vi "MOKE_Teperature and FIeld Sweep_1022D.vi"() -> ()   [LabVIEW 2022 SP3]
uses:
  <vilib>/Analysis/baseanly.llb/Mean (DBL).vi
  <vilib>/Utility/file.llb/Write Delimited Spreadsheet (DBL).vi
  <vilib>/Analysis/NI_AALBase.lvlib
panel:
  out "Rh1 B/A v F":cluster{dbl[], dbl[]}(graph)
  in  "?":bool
  out "Temperature Status":i32(ring) items=["TemperatureUnknown"=0, "Stable"=1, "Tracking"=2, "Near"=5, "Chasing"=6, "Filling"=7, "Standby"=10, "Disabled"=13, "ImpedanceNotFunction"=14, "TempFailure"=15]
  out "Field Status":i32(ring) items=["MagnetUnknown"=0, "StablePersistent"=1, "WarmingSwitch"=2, "CoolingSwitch"=3, "StableDriven"=4, "Iterating"=5, "Charging"=6, "Discharging"=7, "CurrentError"=8, "MagnetFailure"=15]
  out "Field":dbl
  out "Temperature":dbl
  in  "Initialize":bool
  in  "System Stablization (s)":dbl=0.1 format="%#_13g"
  in  "Low Value (Oe)":dbl=-30000.0
  in  "High Value (Oe)":dbl=30000.0
  in  "Sweep Field Approach":i32(ring) items=["Linear", "NoOvershoot", "Oscillate"]
  in  "Sweep F Rate (Oe/s)":dbl=200.0 format="%#_13g"
  in  "Sweep F mode":i32(ring) items=["Persistent", "Driven"]
  in  "Set Fixed T":dbl=2.0
  in  "Fixed Temperature Approach":i32(ring)=1 items=["FastSettle", "NoOvershoot"]
  in  "FIxed T  Rate (K/min)":dbl=20.0
  out "PhaseA-F":cluster{dbl[], dbl[]}(graph)
  out "RA-F":cluster{dbl[], dbl[]}(graph)
  out "Phaseh1B-F":cluster{dbl[], dbl[]}(graph)
  out "Rh1B-F":cluster{dbl[], dbl[]}(graph)
  out "phase B 2":dbl
  in  "Phase B 2":u16(ring)=3 items=["X", "Y", "R", "Theta", "Frequency", "Noise", "Xh1", "Yh1", "Rh1", "Theta h1", "Xh2", "Yh2", "Rh2", "Theta h2"]
  out "phase A 2":dbl
  in  "Phase A 2":u16(ring)=3 items=["X", "Y", "R", "Theta", "Frequency", "Noise", "Xh1", "Yh1", "Rh1", "Theta h1", "Xh2", "Yh2", "Rh2", "Theta h2"]
  out "para1 Measurement (mV) 2":dbl=1.49013e-07
  in  "F Clear Plot A":bool
  in  "Parameter A 2":u16(ring)=2 items=["X", "Y", "R", "Theta", "Frequency", "Noise", "Xh1", "Yh1", "Rh1", "Theta h1", "Xh2", "Yh2", "Rh2", "Theta h2"]
  out "para2 Measurement (uV) 2":dbl=1.49013e-07
  in  "F Clear Plot B":bool
  in  "Parameter B 2":u16(ring)=2 items=["X", "Y", "R", "Theta", "Frequency", "Noise", "Xh1", "Yh1", "Rh1", "Theta h1", "Xh2", "Yh2", "Rh2", "Theta h2"]
  out "Field Setting":dbl format="%#_13g"
  out "Fixed Temperature":dbl
  out "Measured Field":dbl
  out "Field Status":i32(ring) items=["MagnetUnknown"=0, "StablePersistent"=1, "WarmingSwitch"=2, "CoolingSwitch"=3, "StableDriven"=4, "Iterating"=5, "Charging"=6, "Discharging"=7, "CurrentError"=8, "MagnetFailure"=15]
  out "Temperature Status":i32(ring) items=["TemperatureUnknown"=0, "Stable"=1, "Tracking"=2, "Near"=5, "Chasing"=6, "Filling"=7, "Standby"=10, "Disabled"=13, "ImpedanceNotFunction"=14, "TempFailure"=15]
  out "Measuring F":bool
  in  "Step(Oe)":i32=2000
  out "F loop run":i32
  out "Temperature Status":i32(ring) items=["TemperatureUnknown"=0, "Stable"=1, "Tracking"=2, "Near"=5, "Chasing"=6, "Filling"=7, "Standby"=10, "Disabled"=13, "ImpedanceNotFunction"=14, "TempFailure"=15]
  out "Field Status":i32(ring) items=["MagnetUnknown"=0, "StablePersistent"=1, "WarmingSwitch"=2, "CoolingSwitch"=3, "StableDriven"=4, "Iterating"=5, "Charging"=6, "Discharging"=7, "CurrentError"=8, "MagnetFailure"=15]
  out "Fixed Field":dbl
  out "Measured Temperature":dbl
  in  "Delay(T/F)":dbl=3000.0
  in  "Set FIxed F (Oe)":dbl format="%#_13g"
  in  "Fixed Field Approach":i32(ring) items=["Linear", "NoOvershoot", "Oscillate"]
  in  "FIxed F Rate (Oe/s)":dbl=100.0 format="%#_13g"
  in  "Fixed F mode":i32(ring) items=["Persistent", "Driven"]
  in  "Sweep Temperature Approach":i32(ring)=1 items=["FastSettle", "NoOvershoot"]
  in  "Sweep T  Rate (K/min)":dbl=10.0
  in  "Sweep T/F":bool
  in  "Remote":bool=TRUE
  in  "IP Address":string="169.254.170.239"
  out "Measuring T":bool
  in  "A Sine Output Amplitude (V)":sgl=0.1
  in  "path (folder + filename)":string="C:\\Users\\Public\\OneDrive\\Desktop\\MOKE program\\sweep files"
  in  "LOCKIN address":refnum<visa-resource-name>="COM3"
  out "PhaseA-T":cluster{dbl[], dbl[]}(graph)
  out "RA-T":cluster{dbl[], dbl[]}(graph)
  out "Phaseh1-T":cluster{dbl[], dbl[]}(graph)
  out "Rh1B-T":cluster{dbl[], dbl[]}(graph)
  out "phase B":dbl
  in  "Phase B":u16(ring)=9 items=["X", "Y", "R", "Theta", "Frequency", "Noise", "Xh1", "Yh1", "Rh1", "Theta h1", "Xh2", "Yh2", "Rh2", "Theta h2"]
  out "phase A":dbl
  in  "Phase A":u16(ring)=3 items=["X", "Y", "R", "Theta", "Frequency", "Noise", "Xh1", "Yh1", "Rh1", "Theta h1", "Xh2", "Yh2", "Rh2", "Theta h2"]
  out "para1 Measurement (mV)":dbl=1.49013e-07
  in  "T Clear Plot A":bool
  in  "Parameter A":u16(ring)=2 items=["X", "Y", "R", "Theta", "Frequency", "Noise", "Xh1", "Yh1", "Rh1", "Theta h1", "Xh2", "Yh2", "Rh2", "Theta h2"]
  out "para2 Measurement (uV)":dbl=1.49013e-07
  in  "T Clear Plot B":bool
  in  "Parameter B":u16(ring)=8 items=["X", "Y", "R", "Theta", "Frequency", "Noise", "Xh1", "Yh1", "Rh1", "Theta h1", "Xh2", "Yh2", "Rh2", "Theta h2"]
  out "Temperature Setting":dbl format="%#_13g"
  in  "Save data or not":bool=TRUE
  in  "Step(K)":i32=10
  out "T loop run":i32
  in  "B frequency":dbl=267.7 format="%#_13g"
  in  "B Input Connection (0: Single-Ended)":u16(ring)=1 items=["Single-Ended Voltage", "Differential Voltage", "1 MOhm Current Gain", "100 MOhm Current Gain"]
  in  "B harmonic 1":u8=2
  in  "B harmonic 2":u8=3
  in  "B reference Manual Phase":dbl=-59.75
  in  "auto phase B":bool=TRUE
  in  "B Sample time (s)":dbl=0.001 min=0.001 max=100.0 step=0.001
  in  "B Sensitivity":u16(ring)=20 items=["1 nV/fA", "2 nV/fA", "5 nV/fA", "10 nV/fA", "20 nV/fA", "50 nV/fA", "100 nV/fA", "200 nV/fA", "500 nV/fA", "1 uV/pA", "2 uV/pA", "5 uV/pA", "10 uV/pA", "20 uV/pA", "50 uV/pA", "100 uV/pA", "200 uV/pA", "500 uV/pA", "1 mV/nA", "2 mV/nA", "5 mV/nA", "10 mV/nA", "20 mV/nA", "50 mV/nA", "100 mV/nA", "200 mV/nA", "500 mV/nA", "1 V/uA"]
  in  "Enable Sync Filter B (open when f<200Hz)":bool
  in  "B Time Constant":u8(ring)=9 items=["10 us", "30 us", "100 us", "300 us", "1 ms", "3 ms", "10 ms", "30 ms", "100 ms", "300 ms", "1 s", "3 s", "10 s", "30 s", "100 s", "300 s", "1 ks", "3 ks"]
  in  "B Reference Source":u8(ring) items=["External", "Internal", "Internal Sweep", "Channel-A"]
  in  "B Low Pass Filter Slope":u8(ring)=2 items=["6 dB/oct", "12 dB/oct", "18 db/oct", "24 dB/oct"]
  in  "A frequency":dbl=267.7 format="%#_13g"
  in  "A Input Connection (0: Single-Ended)":u16(ring)=1 items=["Single-Ended Voltage", "Differential Voltage", "1 MOhm Current Gain", "100 MOhm Current Gain"]
  in  "A harmonic 1":u8=2
  in  "A harmonic 2":u8=3
  in  "A reference Manual Phase":dbl=-59.75
  in  "auto phase A":bool=TRUE
  in  "A Reference Source":u8(ring)=1 items=["External", "Internal", "Internal Sweep"]
  in  "A Sample time (s)":dbl=0.001 min=0.001 max=100.0 step=0.001
  in  "A Time Constant":u8(ring)=9 items=["10 us", "30 us", "100 us", "300 us", "1 ms", "3 ms", "10 ms", "30 ms", "100 ms", "300 ms", "1 s", "3 s", "10 s", "30 s", "100 s", "300 s", "1 ks", "3 ks"]
  in  "Enable Sync Filter A (open when f<200Hz)":bool
  in  "A Sensitivity":u16(ring)=20 items=["1 nV/fA", "2 nV/fA", "5 nV/fA", "10 nV/fA", "20 nV/fA", "50 nV/fA", "100 nV/fA", "200 nV/fA", "500 nV/fA", "1 uV/pA", "2 uV/pA", "5 uV/pA", "10 uV/pA", "20 uV/pA", "50 uV/pA", "100 uV/pA", "200 uV/pA", "500 uV/pA", "1 mV/nA", "2 mV/nA", "5 mV/nA", "10 mV/nA", "20 mV/nA", "50 mV/nA", "100 mV/nA", "200 mV/nA", "500 mV/nA", "1 V/uA"]
  in  "A Low Pass Filter Slope":u8(ring)=2 items=["6 dB/oct", "12 dB/oct", "18 db/oct", "24 dB/oct"]
  in  "stabilization(S)":dbl=0.1 format="%#_13g"
  in  "High Value (K)":dbl=300.0
  in  "Low Value (K)":dbl=2.0
  in  "loop #":i32=1
  # "Status"
  # "Lock-in Setting"
  # "Channel A"
  # "Channel B"
  # "Sweep F Mesurement"
  # "Temprature and Field Setting"
  # "Sweep T Mesurement"
  # "Sweep F"
  # "Sweep T"
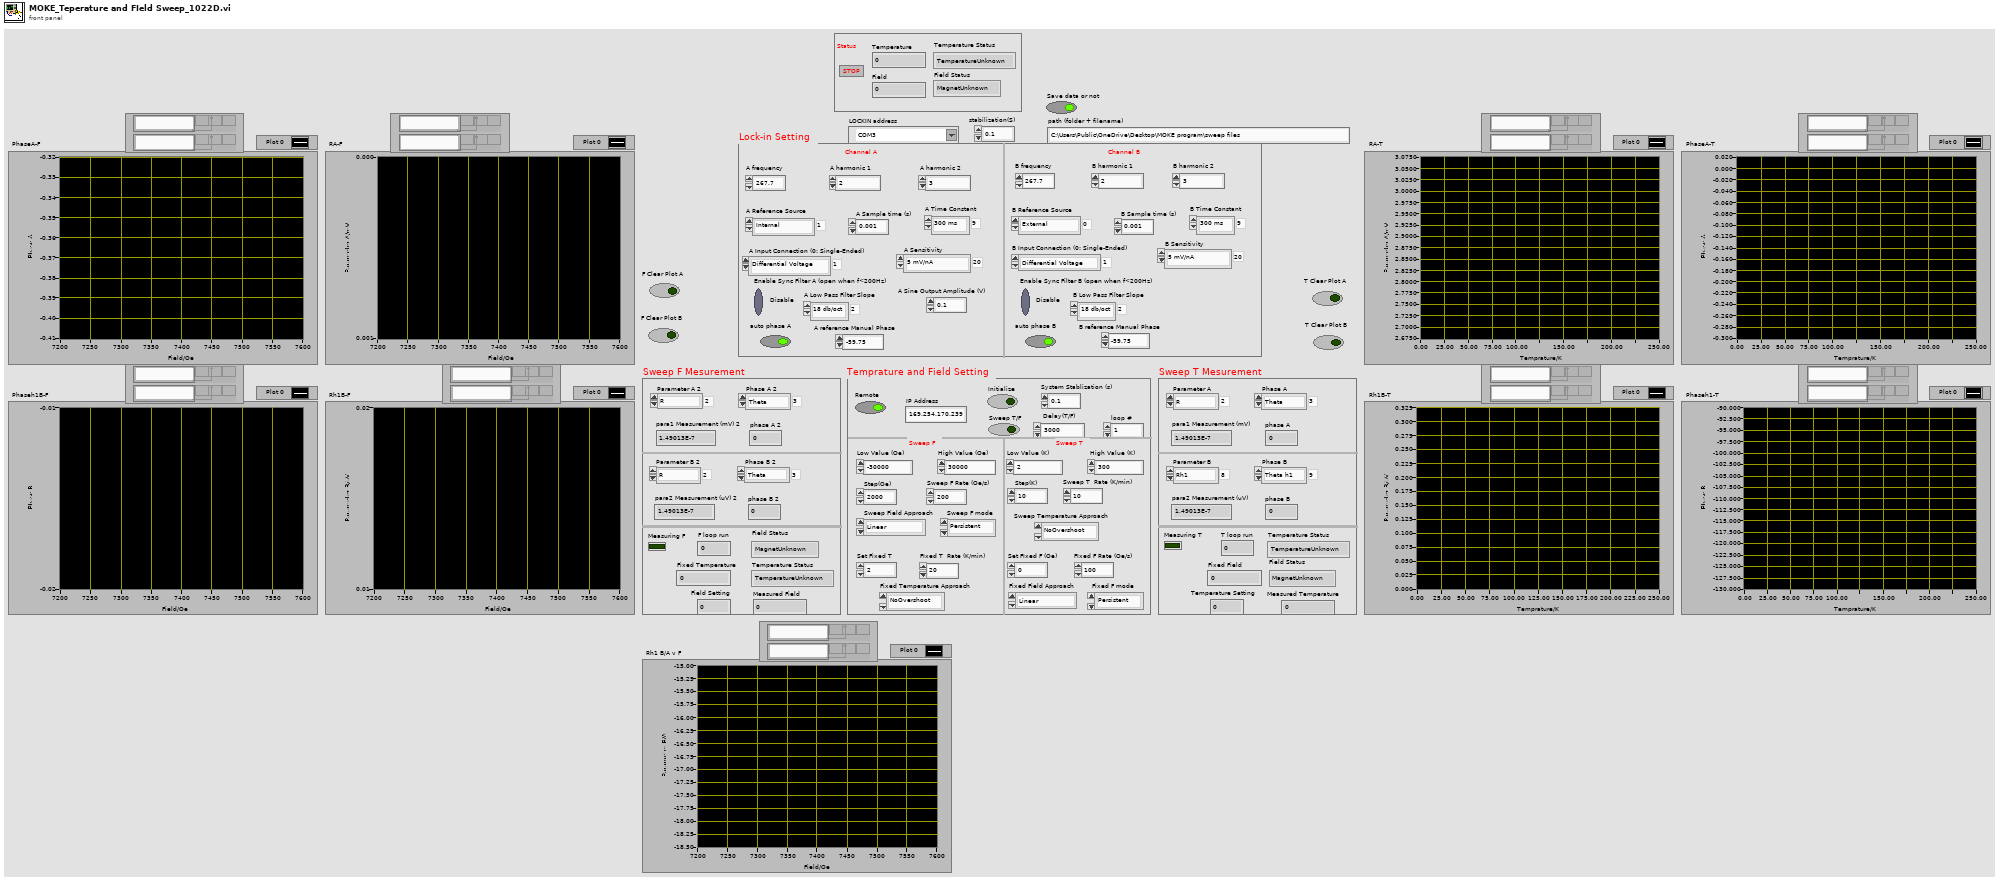
[diagram p1: front panel]
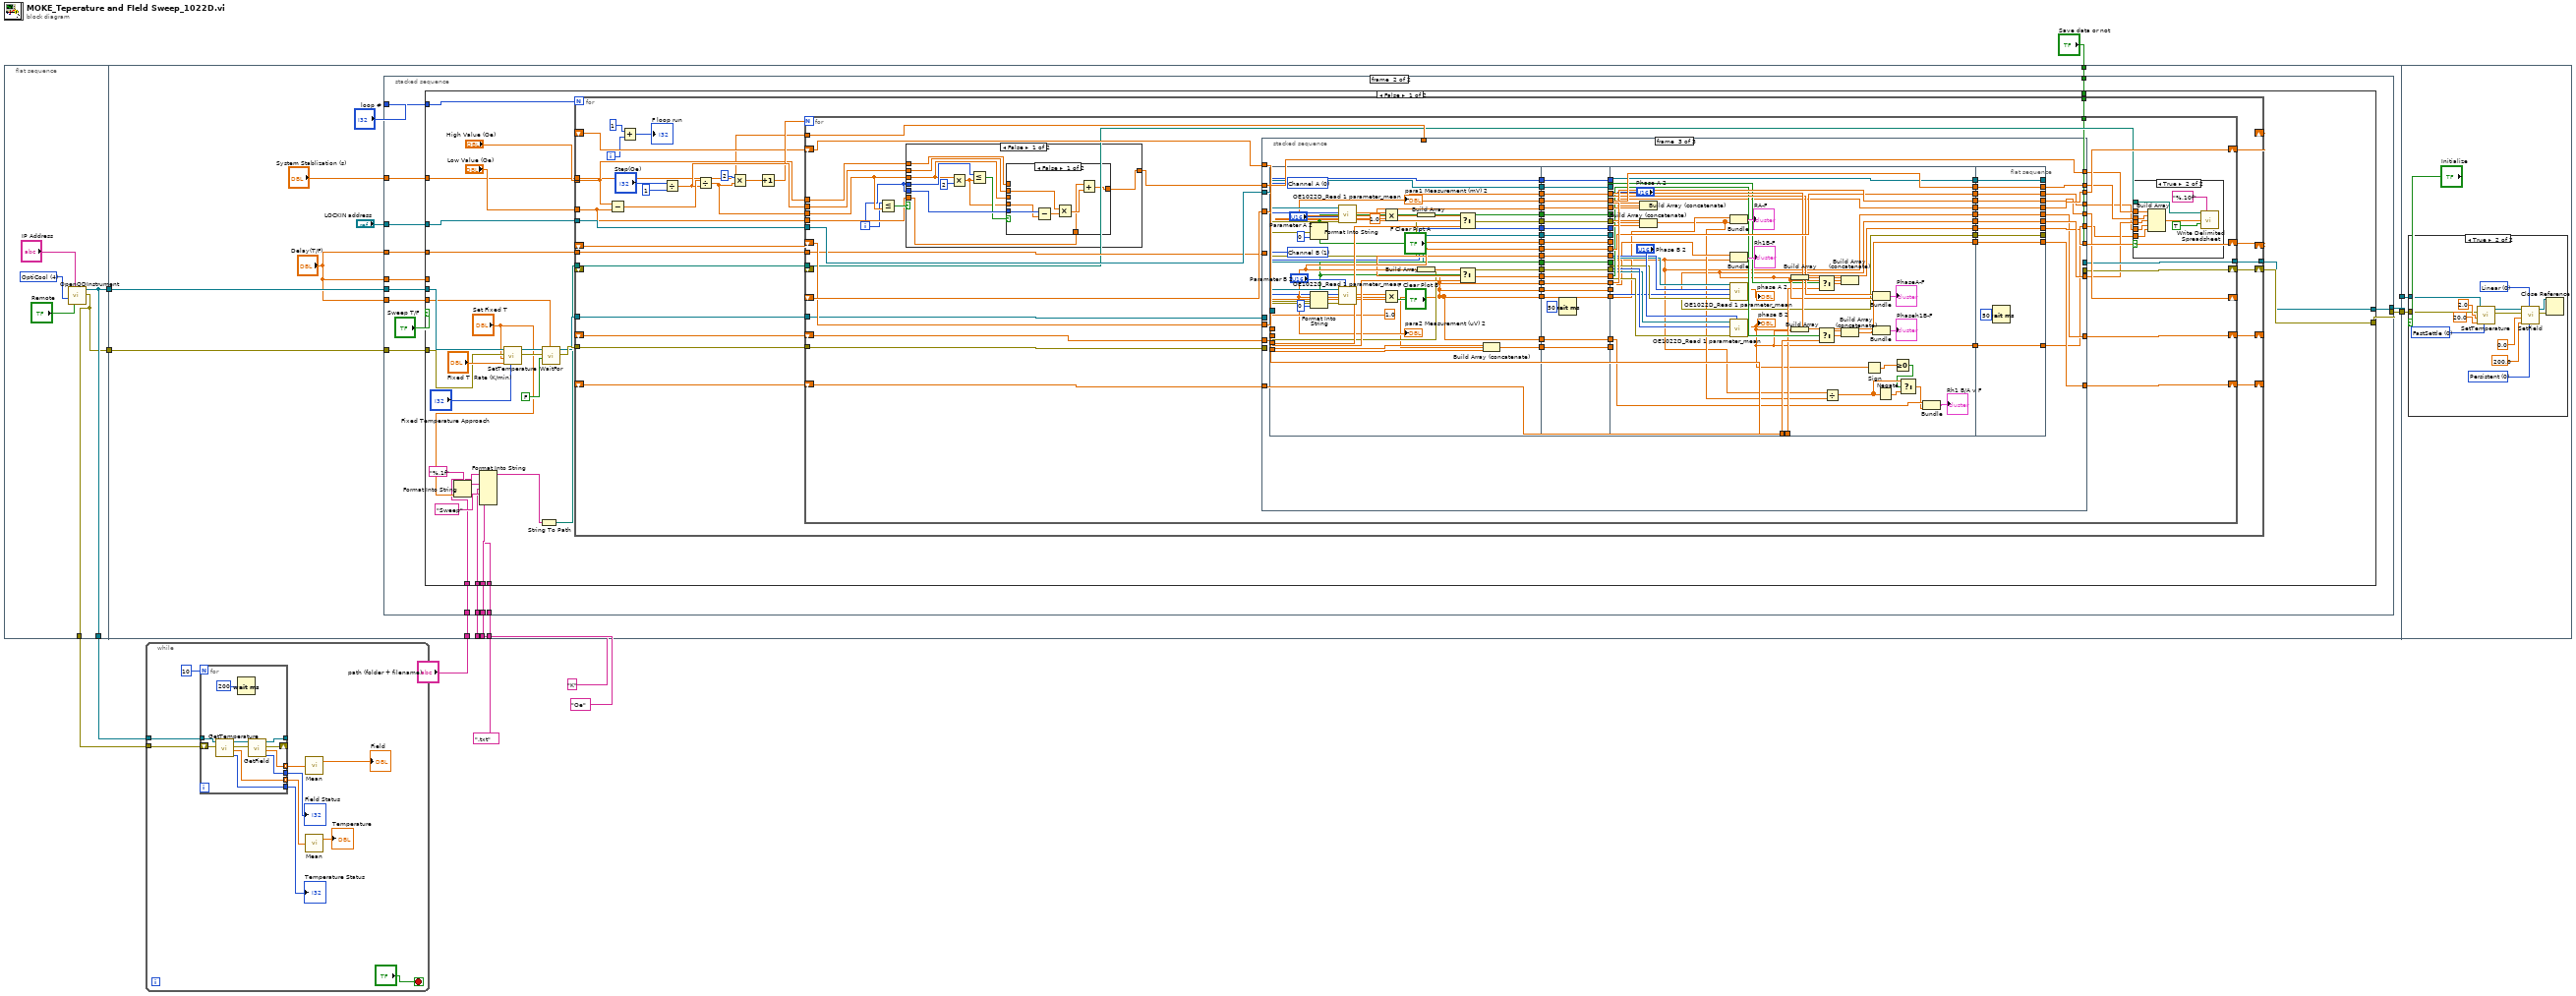
[diagram p0: block diagram]
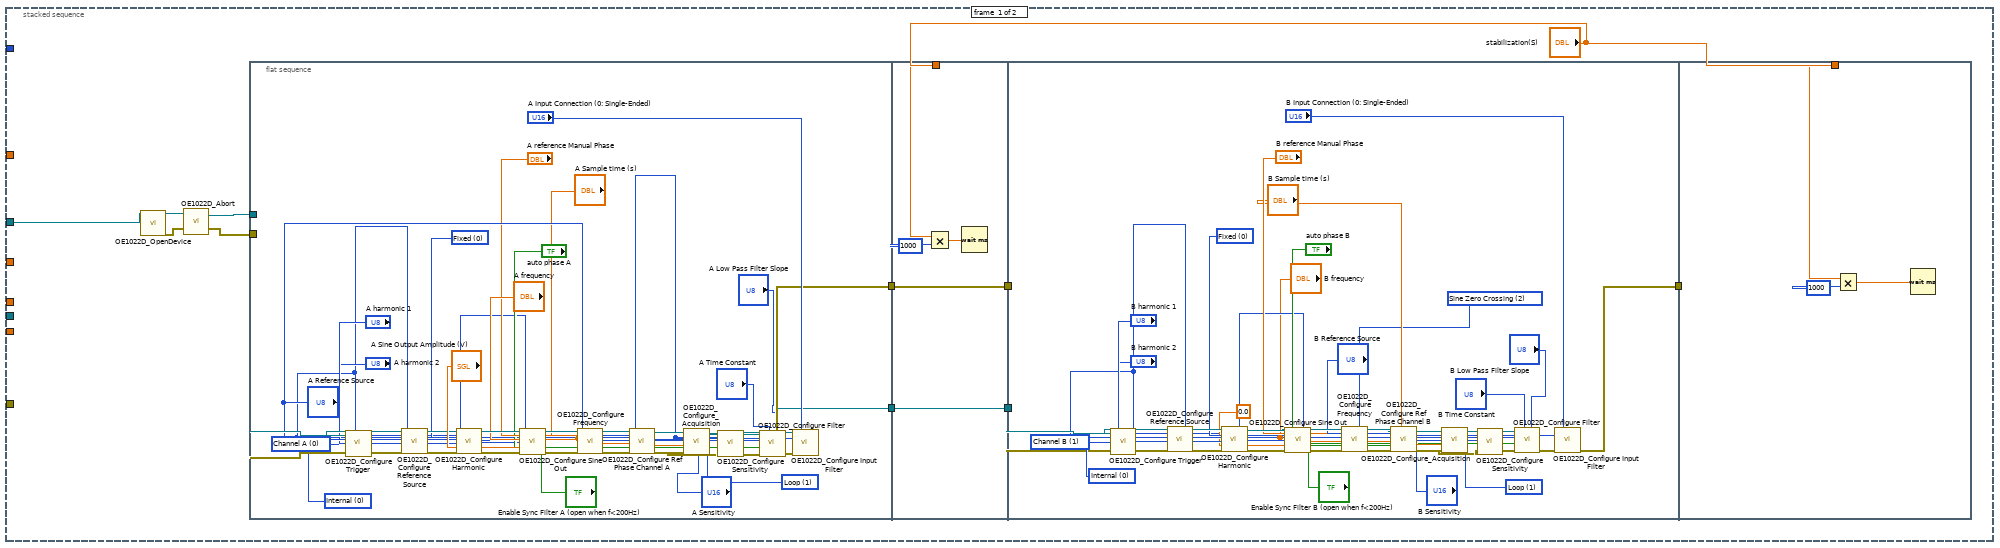
[diagram p2: hidden frame]
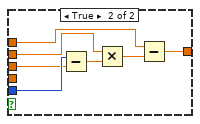
[diagram p4: hidden frame]
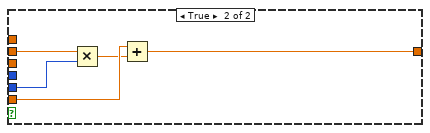
[diagram p5: hidden frame]
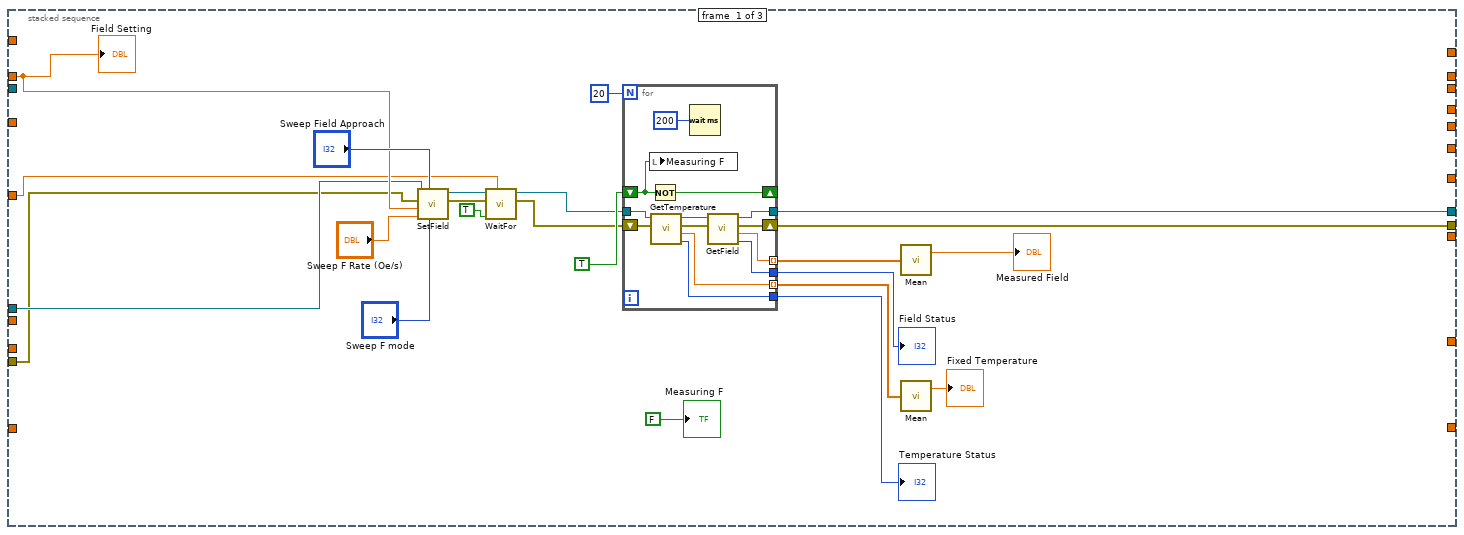
[diagram p6: hidden frame]
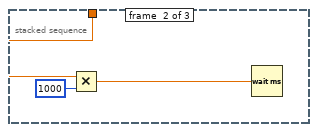
[diagram p7: hidden frame]
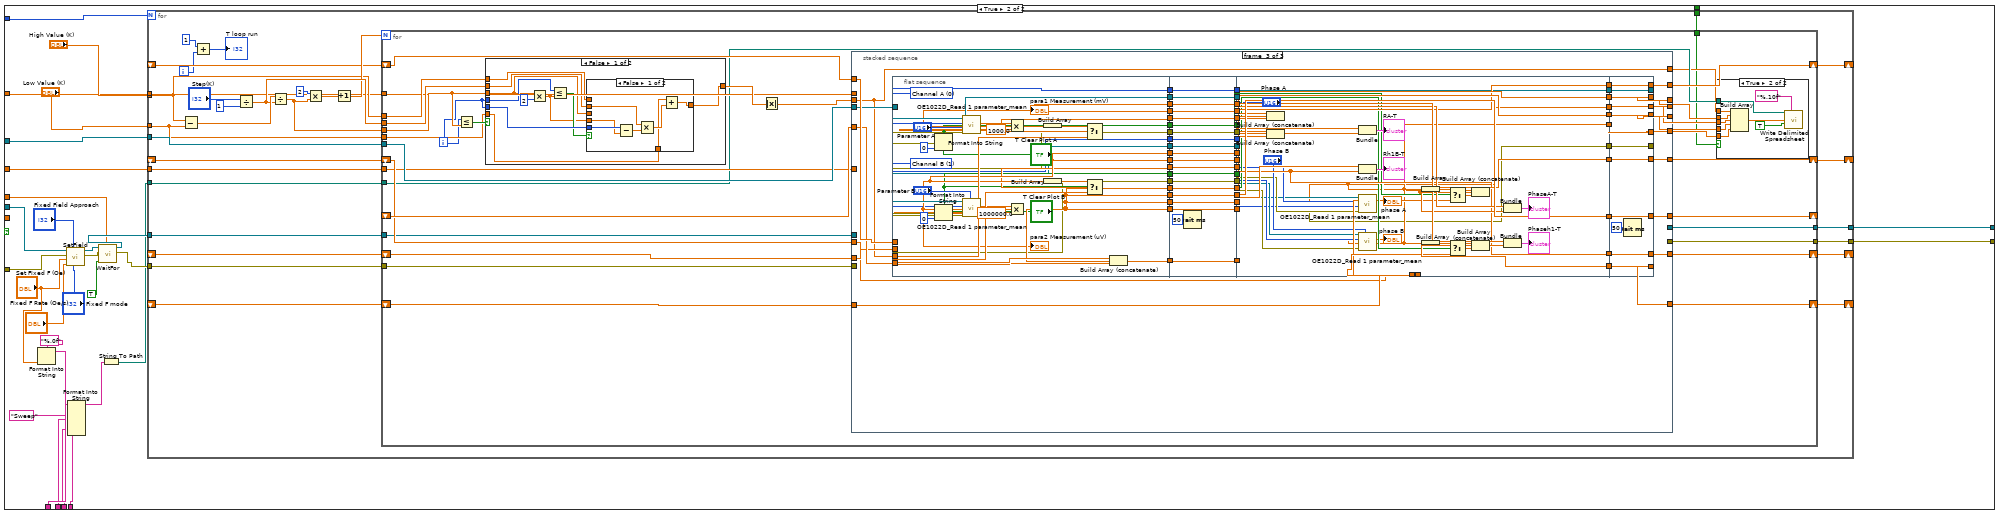
[diagram p8: hidden frame]
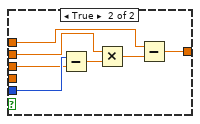
[diagram p10: hidden frame]
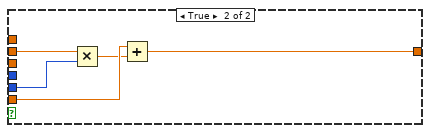
[diagram p11: hidden frame]
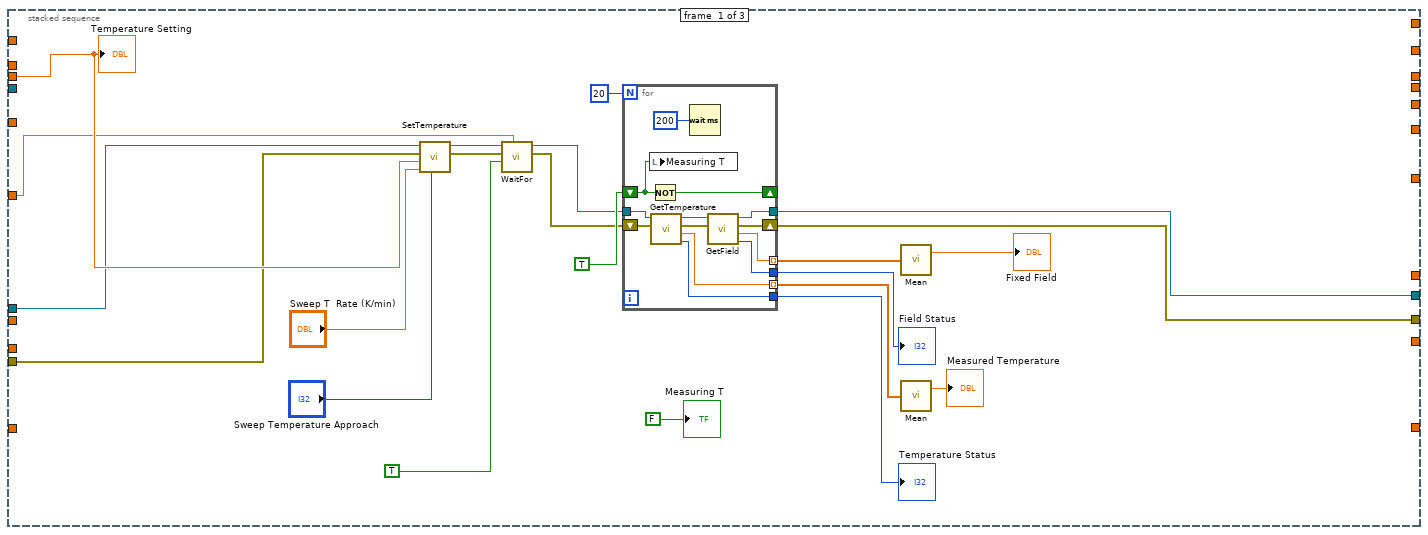
[diagram p12: hidden frame]
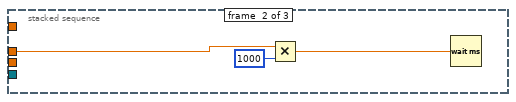
[diagram p13: hidden frame]
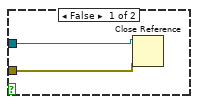
[diagram p14: hidden frame]
diagram:
  n1 = flat-sequence {
    tunnel: [w13] -> w11
    tunnel: [w12] -> w10
    tunnel: [w13] -> w3
    tunnel: [w12] -> w2
    tunnel: w11 -> [w27]
    tunnel: w10 -> [w26]
    tunnel: "path (folder + filename)" -> [w24]
    tunnel: "Oe" -> [w23]
    tunnel: "K" -> [w22]
    tunnel: ".txt" -> [w21]
    tunnel: [w19] -> w5
    tunnel: [w18] -> w4
    tunnel: "Save data or not" -> [w17]
    tunnel: w5 -> [w819]
    tunnel: w4 -> [w818]
    frame #0 {
      w14 = 4 items=["PPMS", "VersaLab", "DynaCool", "SVSM", "OptiCool"] ("InstrumentType")
      n2 = call "OpenQDInstrument.vi"("Remote"="Remote", "IP Address"="IP Address", "InstrumentType"=w14) -> ("error out"=w12:errorcluster, "Instrument Ref"=w13:refnum<k24>)  [unwired: 5 in]
    }
    frame #1 {
      n3 = stacked-sequence {
        tunnel: "LOCKIN address" -> [w32 w141]
        tunnel: "loop #" -> [_ w140]
        tunnel: w27 -> [_ w138]
        tunnel: w26 -> [_ w137]
        tunnel: "Delay(T/F)" -> [_ w136]
        tunnel: "Delay(T/F)" -> [_ w135]
        tunnel: "Delay(T/F)" -> [_ w134]
        tunnel: w24 -> [_ w133]
        tunnel: w23 -> [_ w132]
        tunnel: w22 -> [_ w131]
        tunnel: w21 -> [_ w130]
        tunnel: "System Stablization (s)" -> [_ w129]
        tunnel: [_ w128] -> w19
        tunnel: [_ w127] -> w18
        tunnel: w17 -> [_ w126]
        frame #0 {
          n4 = call "OE1022D_OpenDevice.vi"("VISA resource name"=w32) -> ("VISA资源名称输出"=w31:refnum<visa-resource-name>, "错误输出"=w33:errorcluster)  [unwired: 17 in]
          n5 = call "OE1022D_Abort.vi"("error in (no error)"=w33, "VISA resource name"=w31) -> ("error out"=w38:errorcluster, "VISA resource name out"=w39:refnum<visa-resource-name>)
          n6 = flat-sequence {
            tunnel: w39 -> [w79]
            tunnel: [w67] -> w37
            tunnel: w38 -> [w78]
            tunnel: [w55] -> w35
            tunnel: w37 -> [w84]
            tunnel: [w84] -> w36
            tunnel: w35 -> [w83]
            tunnel: [w83] -> w34
            tunnel: "stabilization(S)" -> [w80]
            tunnel: w36 -> [w105]
            tunnel: [w104] -> w40
            tunnel: w34 -> [w103]
            tunnel: w40 -> [_]
            tunnel: "stabilization(S)" -> [w123]
            frame #0 {
              w41 = u8 1 items=["Single", "Loop"] ("Sample Mode (Single/Loop)")
              w54 = u8 0 items=["Fixed", "Linear", "Log"] ("SineOut Mode")
              w56 = u16 0 items=["Internal", "External"] ("Trigger Source (0: Internal)")
              w45 = u8 0 items=["Channel A", "Channel B"] ("OE1022D A/B")
              n7 = call "OE1022D_Configure Trigger.vi"("Trigger Source (0: Internal)"=w56, "error in (no error)   2"=w78, "OE1022D A/B"=w45, "VISA resource name   2"=w79) -> ("error out   2"=w72:errorcluster, "VISA resource name out   2"=w73:refnum<visa-resource-name>)
              n8 = call "OE1022D_Configure Reference Source.vi"("VISA resource name"=w73, "OE1022D A/B"=w45, "Reference Source"="A Reference Source", "error in (no error)"=w72) -> ("VISA resource name out"=w71:refnum<visa-resource-name>, "error out"=w69:errorcluster)  [unwired: 14 in]
              n9 = call "OE1022D_Configure Harmonic.vi"("VISA resource name"=w71, "OE1022D A/B"=w45, "Harmonic 1"="A harmonic 1", "Harmonic 2"="A harmonic 2", "error in (no error)"=w69) -> ("VISA resource name out"=w70:refnum<visa-resource-name>, "error out"=w68:errorcluster)  [unwired: 13 in]
              n10 = call "OE1022D_Configure Sine Out.vi"("VISA resource name"=w70, "SineOut Mode"=w54, "OE1022D A/B"=w45, "Sine Output Amplitude (V)"="A Sine Output Amplitude (V)", "error in (no error)"=w68) -> ("VISA resource name out"=w76:refnum<visa-resource-name>, "error out"=w75:errorcluster)  [unwired: 9 in]
              n11 = call "OE1022D_Configure Frequency.vi"("VISA resource name"=w76, "OE1022D A/B"=w45, "Internal Frequency(Hz)"="A frequency", "error in (no error)"=w75) -> ("VISA resource name out"=w66:refnum<visa-resource-name>, "error out"=w63:errorcluster)  [unwired: 14 in]
              n12 = call "OE1022D_Configure Ref Phase Channel A.vi"("VISA resource name"=w66, "Reference Source"="A Reference Source", "Internal Frequency(Hz)"="A frequency", "Auto Phase (T: Enabled)"="auto phase A", "error in (no error)"=w63, "Manual Phase  (degree)"="A reference Manual Phase") -> ("VISA resource name out"=w65:refnum<visa-resource-name>, "error out"=w64:errorcluster)  [unwired: 12 in]
              n13 = call "OE1022D_Configure_Acquisition.vi"("VISA resource name"=w65, "OE1022D A/B"=w45, "Sample time (s)"="A Sample time (s)", "error in (no error)"=w64, "Sample Mode (Single/Loop)"=w41) -> ("VISA resource name out"=w48:refnum<visa-resource-name>, "error out"=w47:errorcluster)  [unwired: 3 in]
              n14 = call "OE1022D_Configure Sensitivity.vi"("VISA resource name"=w48, "OE1022D A/B"=w45, "Sensitivity"="A Sensitivity", "error in (no error)"=w47) -> ("VISA resource name out"=w52:refnum<visa-resource-name>, "error out"=w51:errorcluster)  [unwired: 14 in]
              n15 = call "OE1022D_Configure Filter.vi"("Low Pass Filter Slope (1: 12dB/oct)"="A Low Pass Filter Slope", "Time Constant (8: 100ms)"="A Time Constant", "error in (no error)"=w51, "Enable Sync Filter (F: Disable)"="Enable Sync Filter A (open when f<200Hz)", "OE1022D A/B"=w45, "VISA resource name"=w52) -> ("error out"=w49:errorcluster, "VISA resource name out"=w50:refnum<visa-resource-name>)  [unwired: 4 in]
              n16 = call "OE1022D_Configure Input Filter.vi"("VISA resource name"=w50, "Input Source"="A Input Connection (0: Single-Ended)", "OE1022D A/B"=w45, "error in (no error)"=w49) -> ("VISA resource name out"=w55:refnum<visa-resource-name>, "error out"=w67:errorcluster)  [unwired: 10 in]
            }
            frame #1 {
              n17 = Multiply(x=w80, y=1000) -> (x*y=w82:dbl)
              n18 = Wait (ms)(milliseconds to wait=w82) -> ()  [unwired: 1 out]
            }
            frame #2 {
              w85 = u8 1 items=["Single", "Loop"] ("Sample Mode (Single/Loop)")
              w87 = u8 2 items=["TTL Pos", "TTL Neg", "Sine Zero Crossing"] ("External Ref Trigger")
              w100 = u8 0 items=["Fixed", "Linear", "Log"] ("SineOut Mode")
              w106 = u16 0 items=["Internal", "External"] ("Trigger Source (0: Internal)")
              w92 = u8 1 items=["Channel A", "Channel B"] ("OE1022D A/B")
              n19 = call "OE1022D_Configure Trigger.vi"("Trigger Source (0: Internal)"=w106, "error in (no error)   2"=w105, "OE1022D A/B"=w92, "VISA resource name   2"=w103) -> ("error out   2"=w118:errorcluster, "VISA resource name out   2"=w119:refnum<visa-resource-name>)
              n20 = call "OE1022D_Configure Reference Source.vi"("VISA resource name"=w119, "OE1022D A/B"=w92, "error in (no error)"=w118) -> ("VISA resource name out"=w117:refnum<visa-resource-name>, "error out"=w115:errorcluster)  [unwired: 15 in]
              n21 = call "OE1022D_Configure Harmonic.vi"("VISA resource name"=w117, "OE1022D A/B"=w92, "Harmonic 1"="B harmonic 1", "Harmonic 2"="B harmonic 2", "error in (no error)"=w115) -> ("VISA resource name out"=w116:refnum<visa-resource-name>, "error out"=w114:errorcluster)  [unwired: 13 in]
              n22 = call "OE1022D_Configure Sine Out.vi"("VISA resource name"=w116, "SineOut Mode"=w100, "OE1022D A/B"=w92, "Sine Output Amplitude (V)"=sgl 0.0, "error in (no error)"=w114) -> ("VISA resource name out"=w121:refnum<visa-resource-name>, "error out"=w120:errorcluster)  [unwired: 9 in]
              n23 = call "OE1022D_Configure Frequency.vi"("VISA resource name"=w121, "OE1022D A/B"=w92, "Internal Frequency(Hz)"="B frequency", "error in (no error)"=w120) -> ("VISA resource name out"=w113:refnum<visa-resource-name>, "error out"=w110:errorcluster)  [unwired: 14 in]
              n24 = call "OE1022D_Configure Ref Phase Channel B.vi"("VISA resource name"=w113, "Reference Source"="B Reference Source", "External Ref Trigger"=w87, "Internal Frequency(Hz)"="B frequency", "Auto Phase (T: Enabled)"="auto phase B", "error in (no error)"=w110, "Manual Phase  (degree)"="B reference Manual Phase") -> ("VISA resource name out"=w112:refnum<visa-resource-name>, "error out"=w111:errorcluster)  [unwired: 11 in]
              n25 = call "OE1022D_Configure_Acquisition.vi"("VISA resource name"=w112, "OE1022D A/B"=w92, "Sample time (s)"="B Sample time (s)", "error in (no error)"=w111, "Sample Mode (Single/Loop)"=w85) -> ("VISA resource name out"=w93:refnum<visa-resource-name>, "error out"=w94:errorcluster)  [unwired: 3 in]
              n26 = call "OE1022D_Configure Sensitivity.vi"("VISA resource name"=w93, "OE1022D A/B"=w92, "Sensitivity"="B Sensitivity", "error in (no error)"=w94) -> ("VISA resource name out"=w97:refnum<visa-resource-name>, "error out"=w96:errorcluster)  [unwired: 14 in]
              n27 = call "OE1022D_Configure Filter.vi"("Low Pass Filter Slope (1: 12dB/oct)"="B Low Pass Filter Slope", "Time Constant (8: 100ms)"="B Time Constant", "error in (no error)"=w96, "Enable Sync Filter (F: Disable)"="Enable Sync Filter B (open when f<200Hz)", "OE1022D A/B"=w92, "VISA resource name"=w97) -> ("error out"=w95:errorcluster)  [unwired: 4 in, 1 out]
              n28 = call "OE1022D_Configure Input Filter.vi"("Input Source"="B Input Connection (0: Single-Ended)", "OE1022D A/B"=w92, "error in (no error)"=w95) -> ("error out"=w104:errorcluster)  [unwired: 11 in, 1 out]
            }
            frame #3 {
              n29 = Multiply(x=w123, y=1000) -> (x*y=w125:dbl)
              n30 = Wait (ms)(milliseconds to wait=w125) -> ()  [unwired: 1 out]
            }
          }
        }
        frame #1 {
          n31 = case shown="False" "Sweep T/F" {
            tunnel: w141 -> [w169 w513]
            tunnel: w140 -> [w170 w512]
            tunnel: w138 -> [w161 w508]
            tunnel: w137 -> [w162 w507]
            tunnel: w136 -> [_ w501]
            tunnel: w135 -> [w168 w500]
            tunnel: w134 -> [w160 _]
            tunnel: w133 -> [w151 w495]
            tunnel: w132 -> [w150 w491]
            tunnel: w131 -> [w149 w492]
            tunnel: w130 -> [w148 w490]
            tunnel: w129 -> [w145 w487]
            tunnel: [w144 w486] -> w128
            tunnel: [w143 w485] -> w127
            tunnel: w126 -> [w142 w484]
            frame False {
              n32 = Format Into String(format string="%.1f", "Set Fixed T") -> (resulting string=w154:string)  [unwired: 2 in, 1 out]
              n33 = Format Into String(initial string=w151, w154, w149, "Sweep", w150, w148) -> (resulting string=w155:string)  [unwired: 2 in, 1 out]
              n34 = call "SetTemperature.vi"("Approach"="Fixed Temperature Approach", "Rate"="FIxed T  Rate (K/min)", "Temperature"="Set Fixed T", "error in (no error)"=w162, "Instrument Ref In"=w161) -> ("error out"=w163:errorcluster, "Instrument Ref Out"=w164:refnum<k24>)  [unwired: 2 in, 1 out]
              n35 = String To Path(string=w155) -> (path=w152:path)
              n36 = call "WaitFor.vi"("Delay"=w160, "Wait For Temperature"=FALSE ("WaitForTemperature"), "error in (no error)"=w163, "Instrument Ref In"=w164) -> ("error out"=w159:errorcluster, "Instrument Ref Out"=w158:refnum<k24>)  [unwired: 6 in]
              n37 = for {
                N: w170 -> [_]
                tunnel: w169 -> [w200]
                tunnel: "Low Value (Oe)" -> [w194]
                tunnel: "High Value (Oe)" -> [w184]
                tunnel: w152 -> [w193]
                shift-right: [w189] -> _
                shift-left: _ -> [w188]
                shift-right: [w183] -> _
                shift-left: _ -> [w182]
                shift-right: [w181] -> _
                shift-left: _ -> [w180]
                shift-right: [w179] -> _
                shift-left: _ -> [w178]
                tunnel: w158 -> [w177]
                tunnel: w159 -> [w176]
                tunnel: w168 -> [w175]
                tunnel: w145 -> [w174]
                shift-right: [w173] -> w144
                shift-left: _ -> [_]
                tunnel: [w172] -> w143
                tunnel: w142 -> [w171]
                i -> [w186]
                n38 = Subtract(x=w184, y=w194) -> (x-y=w196:dbl)
                n39 = Add(x=1, y=w186) -> (x+y=→"F loop run":i32)
                n40 = Divide(x="Step(Oe)", y=1) -> (x/y=w195:dbl)
                n41 = Divide(x=w196, y=w195) -> (x/y=w192:dbl)
                n42 = Multiply(x=2, y=w192) -> (x*y=w191:dbl)
                n43 = Increment(x=w191) -> (x+1=w190:dbl)
                n44 = for {
                  N: w190 -> [_]
                  tunnel: w200 -> [w231]
                  tunnel: w195 -> [w227]
                  shift-right: [w219] -> w189
                  shift-left: w188 -> [w230]
                  tunnel: w192 -> [w225]
                  tunnel: w194 -> [w228]
                  tunnel: w184 -> [w226]
                  tunnel: w193 -> [w207]
                  shift-right: [w218] -> _
                  shift-left: _ -> [w222]
                  shift-right: [w221] -> w183
                  shift-left: w182 -> [w220]
                  shift-right: [w217] -> w181
                  shift-left: w180 -> [w216]
                  shift-right: [w215] -> w179
                  shift-left: w178 -> [w214]
                  tunnel: w177 -> [w213]
                  tunnel: w176 -> [w212]
                  tunnel: w175 -> [w211]
                  tunnel: w174 -> [w210]
                  shift-right: [w209] -> w173
                  shift-left: _ -> [_]
                  tunnel: [w208] -> w172
                  tunnel: w171 -> [w201]
                  i -> [w224]
                  n45 = Less Or Equal?(x=w224, y=w225) -> (x <= y?=w229:bool)
                  n46 = case shown="False" w229 {
                    tunnel: w228 -> [w241 w269]
                    tunnel: w224 -> [w250 w268]
                    tunnel: w227 -> [w249 w267]
                    tunnel: [w247 w265] -> w223
                    tunnel: w226 -> [w248 _]
                    tunnel: w225 -> [w243 _]
                    tunnel: w224 -> [w246 _]
                    frame False {
                      n47 = Multiply(x=w243, y=2) -> (x*y=w242:dbl)
                      n48 = Less Or Equal?(x=w246, y=w242) -> (x <= y?=w244:bool)
                      n49 = case shown="False" w244 {
                        tunnel: w250 -> [w257 w264]
                        tunnel: w249 -> [w255 w262]
                        tunnel: w248 -> [_ w260]
                        tunnel: [w253 w259] -> w247
                        tunnel: w243 -> [_ w258]
                        tunnel: w242 -> [w252 _]
                        tunnel: w241 -> [w251 _]
                        frame False {
                          n50 = Subtract(x=w257, y=w252) -> (x-y=w256:dbl)
                          n51 = Multiply(x=w255, y=w256) -> (x*y=w254:dbl)
                          n52 = Add(x=w251, y=w254) -> (x+y=w253:dbl)
                        }
                        frame True {
                          n53 = Subtract(x=w264, y=w258) -> (x-y=w263:dbl)
                          n54 = Multiply(x=w262, y=w263) -> (x*y=w261:dbl)
                          n55 = Subtract(x=w260, y=w261) -> (x-y=w259:dbl)
                        }
                      }
                    }
                    frame True {
                      n56 = Multiply(x=w267, y=w268) -> (x*y=w266:dbl)
                      n57 = Add(x=w269, y=w266) -> (x+y=w265:dbl)
                    }
                  }
                  n58 = stacked-sequence {
                    tunnel: w231 -> [_ _ w373]
                    tunnel: w223 -> [w275 _ w372]
                    tunnel: w230 -> [_ _ w375]
                    tunnel: [_ _ w374] -> w219
                    tunnel: [_ _ w311] -> w205
                    tunnel: [_ _ w372] -> w206
                    tunnel: [_ _ w371] -> w218
                    tunnel: w222 -> [_ _ w370]
                    tunnel: [_ _ w369] -> w204
                    tunnel: [_ _ w368] -> w221
                    tunnel: w220 -> [_ _ w361]
                    tunnel: [_ _ w367] -> w217
                    tunnel: w216 -> [_ _ w362]
                    tunnel: [_ _ w366] -> w215
                    tunnel: w214 -> [_ _ w365]
                    tunnel: [_ _ w364] -> w202
                    tunnel: [_ _ w363] -> w203
                    tunnel: w213 -> [w274 _ _]
                    tunnel: w212 -> [w273 _ _]
                    tunnel: w211 -> [w272 _ _]
                    tunnel: w210 -> [_ w306 _]
                    tunnel: [w271 _ _] -> w209
                    tunnel: [w270 _ _] -> w208
                    frame #0 {
                      n59 = call "SetField.vi"("Mode"="Sweep F mode", "Approach"="Sweep Field Approach", "Rate"="Sweep F Rate (Oe/s)", "Field"=w275, "error in (no error)"=w273, "Instrument Ref In"=w274) -> ("error out"=w279:errorcluster, "Instrument Ref Out"=w280:refnum<k24>)  [unwired: 1 in, 1 out]
                      n60 = call "WaitFor.vi"("Delay"=w272, "Wait For Field"=TRUE, "error in (no error)"=w279, "Instrument Ref In"=w280) -> ("error out"=w277:errorcluster, "Instrument Ref Out"=w276:refnum<k24>)  [unwired: 6 in]
                      n61 = for {
                        N: 20 -> [_]
                        shift-right: [w305] -> _
                        shift-left: TRUE -> [w303]
                        shift-right: [w300] -> w271
                        shift-left: w277 -> [w302]
                        tunnel: w276 -> [w299]
                        tunnel: [w297] -> w270
                        tunnel: [w294] -> w290
                        tunnel: [w293] -> w289
                        tunnel: [w295] -> w287 mode=indexing
                        tunnel: [w296] -> w288 mode=indexing
                        n62 = local write "Measuring F"(w303) -> ()
                        n63 = Not(x=w303) -> (.not. x?=w305:bool)
                        n64 = call "GetTemperature.vi"("error in (no error)"=w302, "Instrument Ref In"=w299) -> ("Temperature\nStatus"=w293:i32, "Temperature"=w296:dbl, "error out"=w301:errorcluster, "Instrument Ref Out"=w298:refnum<k24>)  [unwired: 3 in, 1 out]
                        n65 = Wait (ms)(milliseconds to wait=u32 200) -> ()  [unwired: 1 out]
                        n66 = call "GetField.vi"("error in (no error)"=w301, "Instrument Ref In"=w298) -> ("Field\nStatus"=w294:i32, "Field"=w295:dbl, "error out"=w300:errorcluster, "Instrument Ref Out"=w297:refnum<k24>)  [unwired: 3 in, 1 out]
                      }
                      "Field Status" <- w290
                      "Temperature Status" <- w289
                      n67 = call-poly <vilib>:"Mean.vi"("X"=w287) -> ("mean"=→"Measured Field":dbl)  [unwired: 1 out]
                      n68 = call-poly <vilib>:"Mean.vi"("X"=w288) -> ("mean"=→"Fixed Temperature":dbl)  [unwired: 1 out]
                      "Field Setting" <- w275
                      "Measuring F" <- FALSE
                    }
                    frame #1 {
                      n69 = Multiply(x=w306, y=1000) -> (x*y=w308:dbl)
                      n70 = Wait (ms)(milliseconds to wait=w308) -> ()  [unwired: 1 out]
                    }
                    frame #2 {
                      n71 = flat-sequence {
                        tunnel: w375 -> [w403]
                        tunnel: w373 -> [w394]
                        tunnel: w372 -> [w402]
                        tunnel: w370 -> [w401]
                        tunnel: w365 -> [w392]
                        tunnel: [w399] -> w360
                        tunnel: [w387] -> w358
                        tunnel: [w376] -> w356
                        tunnel: [w385] -> w354
                        tunnel: [w376] -> w352
                        tunnel: [w376] -> w350
                        tunnel: [w376] -> w348
                        tunnel: [w376] -> w346
                        tunnel: [w387] -> w344
                        tunnel: [w386] -> w342
                        tunnel: [w385] -> w340
                        tunnel: [w384] -> w338
                        tunnel: ["F Clear Plot B"] -> w336
                        tunnel: ["F Clear Plot A"] -> w334
                        tunnel: [w381] -> w332
                        tunnel: [w380] -> w330
                        tunnel: [w379] -> w328
                        tunnel: [w378] -> w326
                        tunnel: [w377] -> w324
                        tunnel: [w376] -> w309
                        tunnel: w360 -> [w426]
                        tunnel: [w426] -> w359
                        tunnel: w358 -> [w425]
                        tunnel: [w425] -> w357
                        tunnel: w356 -> [w424]
                        tunnel: [w424] -> w355
                        tunnel: w354 -> [w423]
                        tunnel: [w423] -> w353
                        tunnel: w352 -> [w422]
                        tunnel: [w422] -> w351
                        tunnel: w350 -> [w421]
                        tunnel: [w421] -> w349
                        tunnel: w348 -> [w420]
                        tunnel: [w420] -> w347
                        tunnel: w346 -> [w419]
                        tunnel: [w419] -> w345
                        tunnel: w344 -> [w418]
                        tunnel: [w418] -> w343
                        tunnel: w342 -> [w417]
                        tunnel: [w417] -> w341
                        tunnel: w340 -> [w416]
                        tunnel: [w416] -> w339
                        tunnel: w338 -> [w415]
                        tunnel: [w415] -> w337
                        tunnel: w336 -> [w414]
                        tunnel: [w414] -> w335
                        tunnel: w334 -> [w413]
                        tunnel: [w413] -> w333
                        tunnel: w332 -> [w412]
                        tunnel: [w412] -> w331
                        tunnel: w330 -> [w411]
                        tunnel: [w411] -> w329
                        tunnel: w328 -> [w410]
                        tunnel: [w410] -> w327
                        tunnel: w326 -> [w409]
                        tunnel: [w409] -> w325
                        tunnel: w324 -> [w408]
                        tunnel: [w408] -> w323
                        tunnel: [w406] -> w310
                        tunnel: w309 -> [w406]
                        tunnel: w359 -> [w442]
                        tunnel: w357 -> [w471]
                        tunnel: w355 -> [w470]
                        tunnel: w353 -> [w469]
                        tunnel: w351 -> [w468]
                        tunnel: w349 -> [w439]
                        tunnel: w347 -> [w438]
                        tunnel: w345 -> [w464]
                        tunnel: w343 -> [w461]
                        tunnel: w341 -> [w460]
                        tunnel: w339 -> [w458]
                        tunnel: w337 -> [w457]
                        tunnel: w362 -> [w456]
                        tunnel: w335 -> [w455]
                        tunnel: w361 -> [w453]
                        tunnel: w333 -> [w452]
                        tunnel: w331 -> [w448]
                        tunnel: w329 -> [w447]
                        tunnel: w327 -> [w446]
                        tunnel: w325 -> [w444]
                        tunnel: w323 -> [w443]
                        tunnel: [w442] -> w322
                        tunnel: [w437] -> w321
                        tunnel: [w471] -> w320
                        tunnel: [w470] -> w319
                        tunnel: [w433] -> w318
                        tunnel: [w441] -> w317
                        tunnel: [w462] -> w316
                        tunnel: [w459] -> w315
                        tunnel: [w436] -> w314
                        tunnel: [w469] -> w313
                        tunnel: [w429] -> w312
                        tunnel: w310 -> [w435]
                        tunnel: [w473] -> w363
                        tunnel: [w474] -> w364
                        tunnel: [w475] -> w366
                        tunnel: [w476] -> w367
                        tunnel: [w477] -> w368
                        tunnel: [w478] -> _
                        tunnel: [w479] -> w369
                        tunnel: [w480] -> w371
                        tunnel: [w481] -> w311
                        tunnel: [w482] -> w374
                        tunnel: [w483] -> _
                        tunnel: w322 -> [w483]
                        tunnel: w321 -> [w482]
                        tunnel: w320 -> [w481]
                        tunnel: w319 -> [w480]
                        tunnel: w318 -> [w479]
                        tunnel: w317 -> [w478]
                        tunnel: w316 -> [w477]
                        tunnel: w315 -> [w476]
                        tunnel: w314 -> [w475]
                        tunnel: w313 -> [w474]
                        tunnel: w312 -> [w473]
                        frame #0 {
                          w380 = u8 1 items=["Channel A", "Channel B"] ("Channel A/B for Parameter1")
                          w377 = u8 0 items=["Channel A", "Channel B"] ("Channel A/B for Parameter1")
                          n72 = Format Into String(0) -> (error out=w400:errorcluster)  [unwired: 3 in, 1 out]
                          n73 = Format Into String(0) -> (error out=w395:errorcluster)  [unwired: 3 in, 1 out]
                          n74 = call "OE1022D_Read 1 parameter_mean.vi"("错误输入（无错误）"=w400, "Parameter"="Parameter A 2", "Channel (0: A)"=w377, "VISA resource name"=w394) -> ("error out"=w378:errorcluster, "Measurement"=w389:dbl, "VISA resource name out"=w399:refnum<visa-resource-name>)  [unwired: 5 in]
                          n75 = call "OE1022D_Read 1 parameter_mean.vi"("Parameter 2"="Parameter B 2", "错误输入（无错误）"=w395, "Channel (0: A)"=w380, "VISA resource name"=w394) -> ("error out"=w381:errorcluster, "Measurement"=w388:dbl, "VISA resource name out"=w379:refnum<visa-resource-name>)  [unwired: 5 in]
                          n76 = Multiply(x=w389, y=1.0) -> (x*y=w387:dbl)
                          "para1 Measurement (mV) 2" <- w387
                          n77 = Multiply(x=w388, y=1.0) -> (x*y=w385:dbl)
                          "para2 Measurement (uV) 2" <- w385
                          n78 = Build Array(w387) -> (w404:dbl[])
                          n79 = Build Array(w385) -> (w396:dbl[])
                          n80 = Select(t=w404, s="F Clear Plot A", f=w403) -> (s? t:f=w386:dbl[])
                          n81 = Select(t=w396, s="F Clear Plot B", f=w392) -> (s? t:f=w384:dbl[])
                          n82 = Build Array (concatenate)(w402, w401) -> (w376:dbl[])
                        }
                        frame #1 {
                          n83 = Wait (ms)(milliseconds to wait=u32 50) -> ()  [unwired: 1 out]
                        }
                        frame #2 {
                          n84 = Build Array (concatenate)(w461, w460) -> (w437:dbl[])
                          n85 = Build Array (concatenate)(w458, w457) -> (w436:dbl[])
                          n86 = Bundle(w438, w437) -> (→"RA-F":cluster{dbl[], dbl[]})  [unwired: 1 in]
                          n87 = Bundle(w439, w436) -> (→"Rh1B-F":cluster{dbl[], dbl[]})  [unwired: 1 in]
                          n88 = call "OE1022D_Read 1 parameter_mean.vi"("错误输入（无错误）"=w444, "Parameter"="Phase A 2", "Channel (0: A)"=w443, "VISA resource name"=w442) -> ("error out"=w441:errorcluster, "Measurement"=w433:dbl)  [unwired: 5 in, 1 out]
                          "phase A 2" <- w433
                          n89 = call "OE1022D_Read 1 parameter_mean.vi"("Parameter 2"="Phase B 2", "错误输入（无错误）"=w448, "Channel (0: A)"=w447, "VISA resource name"=w446) -> ("Measurement"=w429:dbl)  [unwired: 5 in, 2 out]
                          "phase B 2" <- w429
                          n90 = Build Array(w433) -> (w449:dbl[])
                          n91 = Build Array(w429) -> (w450:dbl[])
                          n92 = Select(t=w449, s=w452, f=w453) -> (s? t:f=w451:dbl[])
                          n93 = Select(t=w450, s=w455, f=w456) -> (s? t:f=w454:dbl[])
                          n94 = Divide(x=w436, y=w437) -> (x/y=w430:dbl[])
                          n95 = Build Array (concatenate)(w433, w451) -> (w462:dbl[])
                          n96 = Build Array (concatenate)(w429, w454) -> (w459:dbl[])
                          n97 = Sign(1:w429) -> (0:w427:dbl)
                          n98 = Bundle(w464, w462) -> (→"PhaseA-F":cluster{dbl[], dbl[]})  [unwired: 1 in]
                          n99 = Bundle(w468, w459) -> (→"Phaseh1B-F":cluster{dbl[], dbl[]})  [unwired: 1 in]
                          n100 = Negate(x=w430) -> (-x=w431:dbl[])
                          n101 = Greater Or Equal To 0?(x=w427) -> (x >= 0?=w428:bool)
                          n102 = Select(t=w430, s=w428, f=w431) -> (s? t:f=w432:dbl[])
                          n103 = Bundle(w435, w432) -> (→"Rh1 B/A v F":cluster{dbl[], dbl[]})  [unwired: 1 in]
                        }
                        frame #3 {
                          n104 = Wait (ms)(milliseconds to wait=u32 50) -> ()  [unwired: 1 out]
                        }
                      }
                    }
                  }
                  n105 = case shown="True" w201 {
                    tunnel: w205 -> [_ w235]
                    tunnel: w206 -> [_ w240]
                    tunnel: w207 -> [_ w238]
                    tunnel: w204 -> [_ w234]
                    tunnel: w202 -> [_ w233]
                    tunnel: w203 -> [_ w232]
                    frame False {
                    }
                    frame True {
                      n106 = Build Array(w240, w235, w234, w233, w232) -> (w237:dbl[])
                      n107 = call-poly <vilib>:"Write Delimited Spreadsheet.vi"("file path (dialog if empty)"=w238, "format (%.3f)"="%.10f", "1D data"=w237, "append to file? (new file:F)"=TRUE) -> ()  [unwired: 10 in, 2 out]
                    }
                  }
                }
              }
            }
            frame True {
              n108 = Format Into String(format string="%.0f", "Set FIxed F (Oe)") -> (resulting string=w494:string)  [unwired: 2 in, 1 out]
              n109 = call "SetField.vi"("Mode"="Fixed F mode", "Approach"="Fixed Field Approach", "Rate"="FIxed F Rate (Oe/s)", "Field"="Set FIxed F (Oe)", "error in (no error)"=w507, "Instrument Ref In"=w508) -> ("error out"=w503:errorcluster, "Instrument Ref Out"=w505:refnum<k24>)  [unwired: 1 in, 1 out]
              n110 = Format Into String(initial string=w495, "Sweep", w492, w494, w491, w490) -> (resulting string=w497:string)  [unwired: 2 in, 1 out]
              n111 = call "WaitFor.vi"("Delay"=w501, "Wait For Field"=TRUE, "error in (no error)"=w503, "Instrument Ref In"=w505) -> ("error out"=w504:errorcluster, "Instrument Ref Out"=w506:refnum<k24>)  [unwired: 6 in]
              n112 = String To Path(string=w497) -> (path=w496:path)
              n113 = for {
                N: w512 -> [_]
                tunnel: w513 -> [w543]
                tunnel: "Low Value (K)" -> [w537]
                tunnel: "High Value (K)" -> [w527]
                tunnel: w496 -> [w536]
                shift-right: [w532] -> _
                shift-left: _ -> [w531]
                shift-right: [w526] -> _
                shift-left: _ -> [w525]
                shift-right: [w524] -> _
                shift-left: _ -> [w523]
                shift-right: [w522] -> _
                shift-left: _ -> [w521]
                tunnel: w506 -> [w520]
                tunnel: w504 -> [w519]
                tunnel: w500 -> [w518]
                tunnel: w487 -> [w517]
                tunnel: [w516] -> w486
                tunnel: [w515] -> w485
                tunnel: w484 -> [w514]
                i -> [w529]
                n114 = Subtract(x=w527, y=w537) -> (x-y=w539:dbl)
                n115 = Add(x=1, y=w529) -> (x+y=→"T loop run":i32)
                n116 = Divide(x="Step(K)", y=1) -> (x/y=w538:dbl)
                n117 = Divide(x=w539, y=w538) -> (x/y=w535:dbl)
                n118 = Multiply(x=2, y=w535) -> (x*y=w534:dbl)
                n119 = Increment(x=w534) -> (x+1=w533:dbl)
                n120 = for {
                  N: w533 -> [_]
                  tunnel: w543 -> [w575]
                  tunnel: w538 -> [w571]
                  shift-right: [w562] -> w532
                  shift-left: w531 -> [w574]
                  tunnel: w535 -> [w569]
                  tunnel: w537 -> [w572]
                  tunnel: w527 -> [w570]
                  tunnel: w536 -> [w546]
                  shift-right: [w551] -> _
                  shift-left: _ -> [w565]
                  shift-right: [w564] -> w526
                  shift-left: w525 -> [w563]
                  shift-right: [w561] -> w524
                  shift-left: w523 -> [w560]
                  shift-right: [w559] -> w522
                  shift-left: w521 -> [w558]
                  tunnel: w520 -> [w557]
                  tunnel: w519 -> [w556]
                  tunnel: w518 -> [w555]
                  tunnel: w517 -> [w554]
                  tunnel: [w553] -> w516
                  tunnel: [w552] -> w515
                  tunnel: w514 -> [w544]
                  i -> [w568]
                  n121 = Less Or Equal?(x=w568, y=w569) -> (x <= y?=w573:bool)
                  n122 = case shown="False" w573 {
                    tunnel: w572 -> [w585 w613]
                    tunnel: w568 -> [w594 w612]
                    tunnel: w571 -> [w593 w611]
                    tunnel: [w591 w609] -> w567
                    tunnel: w570 -> [w592 _]
                    tunnel: w569 -> [w587 _]
                    tunnel: w568 -> [w590 _]
                    frame False {
                      n123 = Multiply(x=w587, y=2) -> (x*y=w586:dbl)
                      n124 = Less Or Equal?(x=w590, y=w586) -> (x <= y?=w588:bool)
                      n125 = case shown="False" w588 {
                        tunnel: w594 -> [w601 w608]
                        tunnel: w593 -> [w599 w606]
                        tunnel: w592 -> [_ w604]
                        tunnel: [w597 w603] -> w591
                        tunnel: w587 -> [_ w602]
                        tunnel: w586 -> [w596 _]
                        tunnel: w585 -> [w595 _]
                        frame False {
                          n126 = Subtract(x=w601, y=w596) -> (x-y=w600:dbl)
                          n127 = Multiply(x=w599, y=w600) -> (x*y=w598:dbl)
                          n128 = Add(x=w595, y=w598) -> (x+y=w597:dbl)
                        }
                        frame True {
                          n129 = Subtract(x=w608, y=w602) -> (x-y=w607:dbl)
                          n130 = Multiply(x=w606, y=w607) -> (x*y=w605:dbl)
                          n131 = Subtract(x=w604, y=w605) -> (x-y=w603:dbl)
                        }
                      }
                    }
                    frame True {
                      n132 = Multiply(x=w611, y=w612) -> (x*y=w610:dbl)
                      n133 = Add(x=w613, y=w610) -> (x+y=w609:dbl)
                    }
                  }
                  n134 = Absolute Value(x=w567) -> (abs(x)=w566:dbl)
                  n135 = stacked-sequence {
                    tunnel: w575 -> [_ _ w714]
                    tunnel: w566 -> [w632 _ w652]
                    tunnel: w574 -> [_ _ w716]
                    tunnel: [_ _ w715] -> w562
                    tunnel: [_ _ w713] -> w547
                    tunnel: [_ _ w712] -> w551
                    tunnel: w565 -> [_ _ w711]
                    tunnel: [_ _ w710] -> w548
                    tunnel: [_ _ w709] -> w564
                    tunnel: w563 -> [_ _ w703]
                    tunnel: [_ _ w708] -> w561
                    tunnel: w560 -> [_ _ w704]
                    tunnel: [_ _ w707] -> w559
                    tunnel: w558 -> [_ _ w706]
                    tunnel: [_ _ w653] -> w549
                    tunnel: [_ _ w705] -> w550
                    tunnel: w557 -> [w631 _ _]
                    tunnel: w556 -> [w630 _ _]
                    tunnel: w555 -> [w627 _ _]
                    tunnel: w554 -> [_ w649 _]
                    tunnel: [w615 _ _] -> w553
                    tunnel: [w614 _ _] -> w552
                    tunnel: [_ _ w652] -> w545
                    frame #0 {
                      n136 = call "SetTemperature.vi"("Approach"="Sweep Temperature Approach", "Rate"="Sweep T  Rate (K/min)", "Temperature"=w632, "error in (no error)"=w630, "Instrument Ref In"=w631) -> ("error out"=w628:errorcluster, "Instrument Ref Out"=w629:refnum<k24>)  [unwired: 2 in, 1 out]
                      n137 = call "WaitFor.vi"("Delay"=w627, "Wait For Temperature"=TRUE ("WaitForTemperature"), "error in (no error)"=w628, "Instrument Ref In"=w629) -> ("error out"=w618:errorcluster, "Instrument Ref Out"=w617:refnum<k24>)  [unwired: 6 in]
                      n138 = for {
                        N: 20 -> [_]
                        shift-right: [w648] -> _
                        shift-left: TRUE -> [w646]
                        shift-right: [w643] -> w615
                        shift-left: w618 -> [w645]
                        tunnel: w617 -> [w642]
                        tunnel: [w640] -> w614
                        tunnel: [w637] -> w624
                        tunnel: [w636] -> w623
                        tunnel: [w638] -> w621 mode=indexing
                        tunnel: [w639] -> w622 mode=indexing
                        n139 = local write "Measuring T"(w646) -> ()
                        n140 = Not(x=w646) -> (.not. x?=w648:bool)
                        n141 = call "GetTemperature.vi"("error in (no error)"=w645, "Instrument Ref In"=w642) -> ("Temperature\nStatus"=w636:i32, "Temperature"=w639:dbl, "error out"=w644:errorcluster, "Instrument Ref Out"=w641:refnum<k24>)  [unwired: 3 in, 1 out]
                        n142 = Wait (ms)(milliseconds to wait=u32 200) -> ()  [unwired: 1 out]
                        n143 = call "GetField.vi"("error in (no error)"=w644, "Instrument Ref In"=w641) -> ("Field\nStatus"=w637:i32, "Field"=w638:dbl, "error out"=w643:errorcluster, "Instrument Ref Out"=w640:refnum<k24>)  [unwired: 3 in, 1 out]
                      }
                      "Field Status" <- w624
                      "Temperature Status" <- w623
                      n144 = call-poly <vilib>:"Mean.vi"("X"=w621) -> ("mean"=→"Fixed Field":dbl)  [unwired: 1 out]
                      n145 = call-poly <vilib>:"Mean.vi"("X"=w622) -> ("mean"=→"Measured Temperature":dbl)  [unwired: 1 out]
                      "Temperature Setting" <- w632
                      "Measuring T" <- FALSE
                    }
                    frame #1 {
                      n146 = Multiply(x=w649, y=1000) -> (x*y=w651:dbl)
                      n147 = Wait (ms)(milliseconds to wait=w651) -> ()  [unwired: 1 out]
                    }
                    frame #2 {
                      n148 = flat-sequence {
                        tunnel: w716 -> [w744]
                        tunnel: w714 -> [w735]
                        tunnel: w652 -> [w743]
                        tunnel: w711 -> [w742]
                        tunnel: w706 -> [w733]
                        tunnel: [w740] -> w702
                        tunnel: [w727] -> w700
                        tunnel: [w728] -> w698
                        tunnel: [w725] -> w696
                        tunnel: [w728] -> w694
                        tunnel: [w728] -> w692
                        tunnel: [w728] -> w690
                        tunnel: [w728] -> w688
                        tunnel: [w727] -> w686
                        tunnel: [w726] -> w684
                        tunnel: [w725] -> w682
                        tunnel: [w724] -> w680
                        tunnel: ["T Clear Plot B"] -> w678
                        tunnel: ["T Clear Plot A"] -> w676
                        tunnel: [w721] -> w674
                        tunnel: [w720] -> w672
                        tunnel: [w719] -> w670
                        tunnel: [w718] -> w668
                        tunnel: [w717] -> w666
                        tunnel: w702 -> [w766]
                        tunnel: [w766] -> w701
                        tunnel: w700 -> [w765]
                        tunnel: [w765] -> w699
                        tunnel: w698 -> [w764]
                        tunnel: [w764] -> w697
                        tunnel: w696 -> [w763]
                        tunnel: [w763] -> w695
                        tunnel: w694 -> [w762]
                        tunnel: [w762] -> w693
                        tunnel: w692 -> [w761]
                        tunnel: [w761] -> w691
                        tunnel: w690 -> [w760]
                        tunnel: [w760] -> w689
                        tunnel: w688 -> [w759]
                        tunnel: [w759] -> w687
                        tunnel: w686 -> [w758]
                        tunnel: [w758] -> w685
                        tunnel: w684 -> [w757]
                        tunnel: [w757] -> w683
                        tunnel: w682 -> [w756]
                        tunnel: [w756] -> w681
                        tunnel: w680 -> [w755]
                        tunnel: [w755] -> w679
                        tunnel: w678 -> [w754]
                        tunnel: [w754] -> w677
                        tunnel: w676 -> [w753]
                        tunnel: [w753] -> w675
                        tunnel: w674 -> [w752]
                        tunnel: [w752] -> w673
                        tunnel: w672 -> [w751]
                        tunnel: [w751] -> w671
                        tunnel: w670 -> [w750]
                        tunnel: [w750] -> w669
                        tunnel: w668 -> [w749]
                        tunnel: [w749] -> w667
                        tunnel: w666 -> [w748]
                        tunnel: [w748] -> w665
                        tunnel: w701 -> [w770]
                        tunnel: w699 -> [w804]
                        tunnel: w697 -> [w803]
                        tunnel: w695 -> [w802]
                        tunnel: w693 -> [w801]
                        tunnel: w691 -> [w799]
                        tunnel: w689 -> [w797]
                        tunnel: w687 -> [w795]
                        tunnel: w685 -> [w792]
                        tunnel: w683 -> [w791]
                        tunnel: w681 -> [w788]
                        tunnel: w679 -> [w787]
                        tunnel: w704 -> [w785]
                        tunnel: w677 -> [w784]
                        tunnel: w703 -> [w782]
                        tunnel: w675 -> [w781]
                        tunnel: w673 -> [w777]
                        tunnel: w671 -> [w776]
                        tunnel: w669 -> [w775]
                        tunnel: w667 -> [w772]
                        tunnel: w665 -> [w771]
                        tunnel: [w770] -> w664
                        tunnel: [w790] -> w663
                        tunnel: [w804] -> w662
                        tunnel: [w803] -> w661
                        tunnel: [w768] -> w660
                        tunnel: [w769] -> w659
                        tunnel: [w793] -> w658
                        tunnel: [w789] -> w657
                        tunnel: [w786] -> w656
                        tunnel: [w802] -> w655
                        tunnel: [w774] -> w654
                        tunnel: [w808] -> w705
                        tunnel: [w809] -> w653
                        tunnel: [w806] -> w707
                        tunnel: [w810] -> w708
                        tunnel: [w811] -> w709
                        tunnel: [w812] -> _
                        tunnel: [w813] -> w710
                        tunnel: [w814] -> w712
                        tunnel: [w815] -> w713
                        tunnel: [w805] -> w715
                        tunnel: [w816] -> _
                        tunnel: w664 -> [w816]
                        tunnel: w663 -> [w805]
                        tunnel: w662 -> [w815]
                        tunnel: w661 -> [w814]
                        tunnel: w660 -> [w813]
                        tunnel: w659 -> [w812]
                        tunnel: w658 -> [w811]
                        tunnel: w657 -> [w810]
                        tunnel: w656 -> [w806]
                        tunnel: w655 -> [w809]
                        tunnel: w654 -> [w808]
                        frame #0 {
                          w720 = u8 1 items=["Channel A", "Channel B"] ("Channel A/B for Parameter1")
                          w717 = u8 0 items=["Channel A", "Channel B"] ("Channel A/B for Parameter1")
                          n149 = Format Into String(0) -> (error out=w741:errorcluster)  [unwired: 3 in, 1 out]
                          n150 = Format Into String(0) -> (error out=w736:errorcluster)  [unwired: 3 in, 1 out]
                          n151 = call "OE1022D_Read 1 parameter_mean.vi"("错误输入（无错误）"=w741, "Parameter"="Parameter A", "Channel (0: A)"=w717, "VISA resource name"=w735) -> ("error out"=w718:errorcluster, "Measurement"=w730:dbl, "VISA resource name out"=w740:refnum<visa-resource-name>)  [unwired: 5 in]
                          n152 = call "OE1022D_Read 1 parameter_mean.vi"("Parameter 2"="Parameter B", "错误输入（无错误）"=w736, "Channel (0: A)"=w720, "VISA resource name"=w735) -> ("error out"=w721:errorcluster, "Measurement"=w729:dbl, "VISA resource name out"=w719:refnum<visa-resource-name>)  [unwired: 5 in]
                          n153 = Multiply(x=w730, y=1000.0) -> (x*y=w727:dbl)
                          "para1 Measurement (mV)" <- w727
                          n154 = Multiply(x=w729, y=1000000.0) -> (x*y=w725:dbl)
                          "para2 Measurement (uV)" <- w725
                          n155 = Build Array(w727) -> (w745:dbl[])
                          n156 = Build Array(w725) -> (w737:dbl[])
                          n157 = Select(t=w745, s="T Clear Plot A", f=w744) -> (s? t:f=w726:dbl[])
                          n158 = Select(t=w737, s="T Clear Plot B", f=w733) -> (s? t:f=w724:dbl[])
                          n159 = Build Array (concatenate)(w743, w742) -> (w728:dbl[])
                        }
                        frame #1 {
                          n160 = Wait (ms)(milliseconds to wait=u32 50) -> ()  [unwired: 1 out]
                        }
                        frame #2 {
                          n161 = Build Array (concatenate)(w792, w791) -> (w790:dbl[])
                          n162 = Build Array (concatenate)(w788, w787) -> (w786:dbl[])
                          n163 = Bundle(w797, w790) -> (→"RA-T":cluster{dbl[], dbl[]})  [unwired: 1 in]
                          n164 = Bundle(w799, w786) -> (→"Rh1B-T":cluster{dbl[], dbl[]})  [unwired: 1 in]
                          n165 = call "OE1022D_Read 1 parameter_mean.vi"("错误输入（无错误）"=w772, "Parameter"="Phase A", "Channel (0: A)"=w771, "VISA resource name"=w770) -> ("error out"=w769:errorcluster, "Measurement"=w768:dbl)  [unwired: 5 in, 1 out]
                          "phase A" <- w768
                          n166 = call "OE1022D_Read 1 parameter_mean.vi"("Parameter 2"="Phase B", "错误输入（无错误）"=w777, "Channel (0: A)"=w776, "VISA resource name"=w775) -> ("Measurement"=w774:dbl)  [unwired: 5 in, 2 out]
                          "phase B" <- w774
                          n167 = Build Array(w768) -> (w778:dbl[])
                          n168 = Build Array(w774) -> (w779:dbl[])
                          n169 = Select(t=w778, s=w781, f=w782) -> (s? t:f=w780:dbl[])
                          n170 = Select(t=w779, s=w784, f=w785) -> (s? t:f=w783:dbl[])
                          n171 = Build Array (concatenate)(w768, w780) -> (w793:dbl[])
                          n172 = Build Array (concatenate)(w774, w783) -> (w789:dbl[])
                          n173 = Bundle(w795, w793) -> (→"PhaseA-T":cluster{dbl[], dbl[]})  [unwired: 1 in]
                          n174 = Bundle(w801, w789) -> (→"Phaseh1-T":cluster{dbl[], dbl[]})  [unwired: 1 in]
                        }
                        frame #3 {
                          n175 = Wait (ms)(milliseconds to wait=u32 50) -> ()  [unwired: 1 out]
                        }
                      }
                    }
                  }
                  n176 = case shown="True" w544 {
                    tunnel: w547 -> [_ w579]
                    tunnel: w545 -> [_ w584]
                    tunnel: w546 -> [_ w582]
                    tunnel: w548 -> [_ w578]
                    tunnel: w549 -> [_ w577]
                    tunnel: w550 -> [_ w576]
                    frame False {
                    }
                    frame True {
                      n177 = Build Array(w584, w579, w578, w577, w576) -> (w581:dbl[])
                      n178 = call-poly <vilib>:"Write Delimited Spreadsheet.vi"("file path (dialog if empty)"=w582, "format (%.3f)"="%.10f", "1D data"=w581, "append to file? (new file:F)"=TRUE) -> ()  [unwired: 10 in, 2 out]
                    }
                  }
                }
              }
            }
          }
        }
      }
    }
    frame #2 {
      n179 = case shown="True" "Initialize" {
        tunnel: w819 -> [w820 w823]
        tunnel: w818 -> [w821 w822]
        frame False {
          n180 = Close Reference(reference=w821, error in (no error)=w820) -> ()  [unwired: 1 out]
        }
        frame True {
          w829 = 0 items=["Linear", "NoOvershoot", "Oscillate"] ("Approach")
          w830 = 0 items=["Persistent", "Driven"] ("Mode")
          w826 = 0 items=["FastSettle", "NoOvershoot"] ("Approach")
          n181 = call "SetTemperature.vi"("Approach"=w826, "Rate"=20.0, "Temperature"=2.0, "error in (no error)"=w823, "Instrument Ref In"=w822) -> ("error out"=w834:errorcluster, "Instrument Ref Out"=w833:refnum<k24>)  [unwired: 2 in, 1 out]
          n182 = call "SetField.vi"("Mode"=w830, "Approach"=w829, "Rate"=200.0, "Field"=0.0, "error in (no error)"=w834, "Instrument Ref In"=w833) -> ("error out"=w831:errorcluster, "Instrument Ref Out"=w832:refnum<k24>)  [unwired: 1 in, 1 out]
          n183 = Close Reference(reference=w832, error in (no error)=w831) -> ()  [unwired: 1 out]
        }
      }
    }
  }
  n184 = while {
    tunnel: w3 -> [w837]
    tunnel: w2 -> [w836]
    stop <- "?" stop-if-true
    n185 = for {
      N: 10 -> [_]
      shift-right: [w852] -> _
      shift-left: w836 -> [w854]
      tunnel: w837 -> [w851]
      tunnel: [w849] -> _
      tunnel: [w846] -> w843
      tunnel: [w845] -> w842
      tunnel: [w847] -> w840 mode=indexing
      tunnel: [w848] -> w841 mode=indexing
      n186 = call "GetTemperature.vi"("error in (no error)"=w854, "Instrument Ref In"=w851) -> ("Temperature\nStatus"=w845:i32, "Temperature"=w848:dbl, "error out"=w853:errorcluster, "Instrument Ref Out"=w850:refnum<k24>)  [unwired: 3 in, 1 out]
      n187 = Wait (ms)(milliseconds to wait=u32 200) -> ()  [unwired: 1 out]
      n188 = call "GetField.vi"("error in (no error)"=w853, "Instrument Ref In"=w850) -> ("Field\nStatus"=w846:i32, "Field"=w847:dbl, "error out"=w852:errorcluster, "Instrument Ref Out"=w849:refnum<k24>)  [unwired: 3 in, 1 out]
    }
    "Field Status" <- w843
    "Temperature Status" <- w842
    n189 = call-poly <vilib>:"Mean.vi"("X"=w840) -> ("mean"=→"Field":dbl)  [unwired: 1 out]
    n190 = call-poly <vilib>:"Mean.vi"("X"=w841) -> ("mean"=→"Temperature":dbl)  [unwired: 1 out]
  }
